vi "Set Manager QueryPlugin Response.vi"(7 "Streaming? (F)":bool, 8 "error in (no error)":errorcluster, 10 "Message Data":T1, 11 "gRPCid in":T14) -> (0 "error out":errorcluster)   [LabVIEW 2021, in "CIF_Manager_server.lvlib" / "Manager.lvclass"]
uses:
  Manager.lvclass
  <vilib>/gRPC/LabVIEW gRPC Library/Shared/grpcId.ctl
  Manager.lvclass/Manager.ctl
  CIF_Manager_server.lvlib
  <vilib>/gRPC/LabVIEW gRPC Library/grpc-lvsupport-release.lvlib
  RPC Messages/cif_common_Status.ctl
  RPC Messages/cif_plugincore_MonitorI64.ctl
  RPC Messages/cif_plugincore_MonitorU64.ctl
  RPC Messages/cif_plugincore_MonitorDoubles.ctl
  RPC Messages/cif_plugincore_Error.ctl
  RPC Messages/cif_common_TimingStats.ctl
  RPC Messages/cif_plugincore_FifoStatistics.ctl
  RPC Messages/cif_plugincore_TimingStatistics.ctl
  RPC Messages/cif_plugincore_StatusData_State.ctl
  RPC Messages/cif_plugincore_StatusData.ctl
  RPC Messages/cif_common_ShortVersion.ctl
  RPC Messages/cif_manager_PluginInfo.ctl
  RPC Messages/cif_manager_PluginInfoResponse.ctl
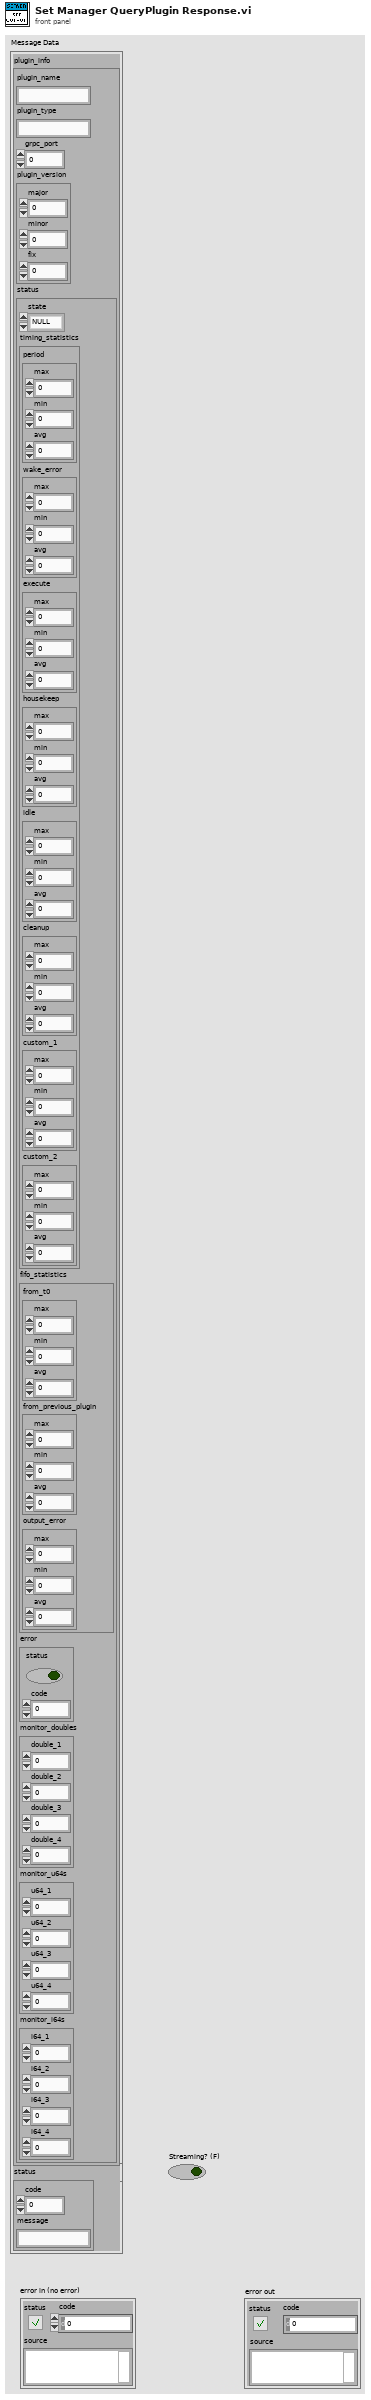
[diagram p1: front panel]
types:
  T1 = typedef "CIF_Manager_server.lvlib/cif_manager_PluginInfoResponse.ctl" = cluster{"plugin_info":T2, "status":T13}
  T2 = typedef "CIF_Manager_server.lvlib/cif_manager_PluginInfo.ctl" = cluster{"plugin_name":string, "plugin_type":string, "grpc_port":i32, "plugin_version":T3, "status":T4}
  T3 = typedef "CIF_Manager_server.lvlib/cif_common_ShortVersion.ctl" = cluster{"major":u32, "minor":u32, "fix":u32}
  T4 = typedef "CIF_Manager_server.lvlib/cif_plugincore_StatusData.ctl" = cluster{"state":T5, "timing_statistics":T6, "fifo_statistics":T8, "error":T9, "monitor_doubles":T10, "monitor_u64s":T11, "monitor_i64s":T12}
  T5 = typedef "CIF_Manager_server.lvlib/cif_plugincore_StatusData_State.ctl" = enum32{"NULL", "CREATING", "LISTENING", "RUNNING", "CLEANINGUP", "DESTROYING"}
  T6 = typedef "CIF_Manager_server.lvlib/cif_plugincore_TimingStatistics.ctl" = cluster{"period":T7, "wake_error":T7, "execute":T7, "housekeep":T7, "idle":T7, "cleanup":T7, "custom_1":T7, "custom_2":T7}
  T7 = typedef "CIF_Manager_server.lvlib/cif_common_TimingStats.ctl" = cluster{"max":i64, "min":i64, "avg":dbl}
  T8 = typedef "CIF_Manager_server.lvlib/cif_plugincore_FifoStatistics.ctl" = cluster{"from_t0":T7, "from_previous_plugin":T7, "output_error":T7}
  T9 = typedef "CIF_Manager_server.lvlib/cif_plugincore_Error.ctl" = cluster{"status":bool, "code":i32}
  T10 = typedef "CIF_Manager_server.lvlib/cif_plugincore_MonitorDoubles.ctl" = cluster{"double_1":dbl, "double_2":dbl, "double_3":dbl, "double_4":dbl}
  T11 = typedef "CIF_Manager_server.lvlib/cif_plugincore_MonitorU64.ctl" = cluster{"u64_1":u64, "u64_2":u64, "u64_3":u64, "u64_4":u64}
  T12 = typedef "CIF_Manager_server.lvlib/cif_plugincore_MonitorI64.ctl" = cluster{"i64_1":i64, "i64_2":i64, "i64_3":i64, "i64_4":i64}
  T13 = typedef "CIF_Manager_server.lvlib/cif_common_Status.ctl" = cluster{"code":i32, "message":string}
  T14 = typedef "grpc-lvsupport-release.lvlib/grpcId.ctl" = u64
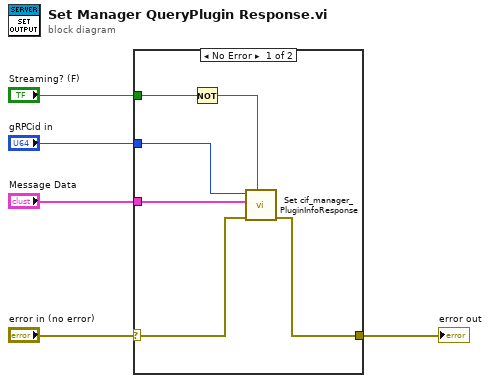
[diagram p0: block diagram]
diagram:
  n1 = case shown="No Error" "error in (no error)" {
    selector: "error in (no error)" -> [w11 w12]
    tunnel: [w9 w12] -> w4
    tunnel: "gRPCid in" -> [w10 _]
    tunnel: "Message Data" -> [w8 _]
    tunnel: "Streaming? (F)" -> [w7 _]
    frame No Error {
      n2 = Not(x=w7) -> (.not. x?=w6:bool)
      n3 = call "Set cif_manager_PluginInfoResponse.vi"("Complete Call (T)"=w6, "error in (no error)"=w11, "package_templatemessage"=w8, "gRPCid"=w10) -> ("error out"=w9:errorcluster)  [unwired: 7 in]
    }
    frame Error {
    }
  }
  "error out" <- w4
